vi "Create From VI Reference.vi"(8 "error in (no error)":errorcluster, 10 "VI":refnum<vi>) -> (0 "error out":errorcluster, 3 "CSM-Helper.lvclass":refnum<class "CSM-Helper.lvclass">)   [LabVIEW 2020, in "CSM-Helper.lvclass"]
uses:
  CSM-Helper.lvclass
  CSM-Helper.lvclass/CSM-Helper.ctl
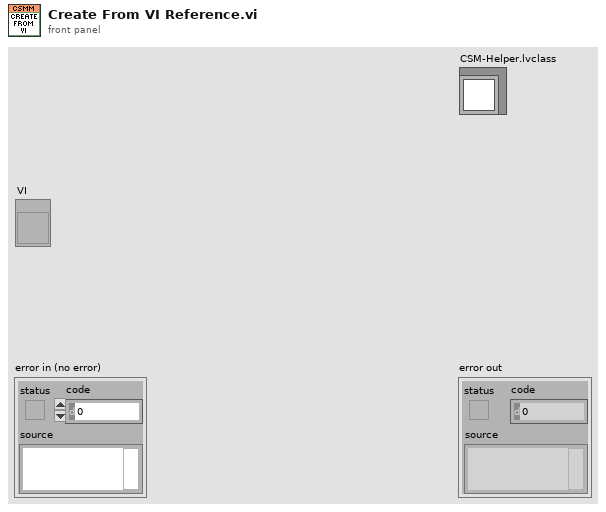
[diagram p1: front panel]
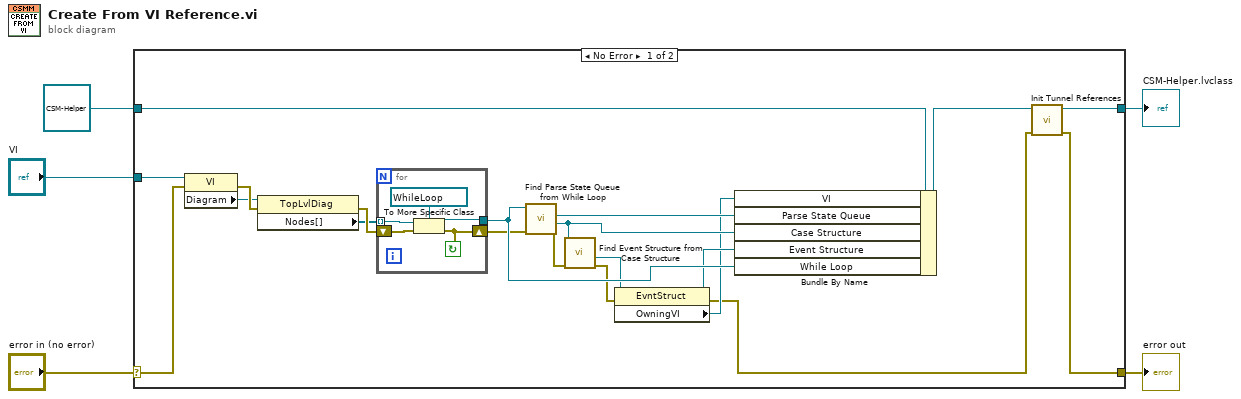
[diagram p0: block diagram]
diagram:
  n1 = case shown="No Error" "error in (no error)" {
    selector: "error in (no error)" -> [w20 w32]
    tunnel: [w6 w32] -> w4
    tunnel: [w8 w31] -> w2
    tunnel: refnum<class "CSM-Helper.lvclass"> refnum ("JKI SM") -> [w19 w31]
    tunnel: "VI" -> [w21 _]
    frame No Error {
      n2 = property class="VI"(reference=w21, error in=w20) -> (error out=w25:errorcluster, "Diagram"=w22:refnum<vi>)  [unwired: 1 out]
      n3 = property class="TopLvlDiag"(reference=w22, error in=w25) -> (error out=w24:errorcluster, "Nodes[]"=w23:refnum<vi>[])  [unwired: 1 out]
      n4 = for {
        tunnel: w23 -> [w29] mode=indexing
        tunnel: [w27] -> w16
        shift-right: [w26] -> w15
        shift-left: w24 -> [w28]
        stop <- w26 continue-if-true
        n5 = To More Specific Class(target class=refnum<vi> refnum ("WLoop Refnum"), reference=w29, error in=w28) -> (specific class reference=w27:refnum<vi>, error out=w26:errorcluster)
      }
      n6 = call "Find Parse State Queue from While Loop.vi"("error in (no error)"=w15, "WhileLoop in"=w16) -> ("error out"=w17:errorcluster, "CaseStructure"=w14:refnum<vi>, "Parse State Queue"=w18:refnum<vi>)  [unwired: 7 in]
      n7 = call "Find Event Structure from Case Structure.vi"("error in (no error)"=w17, "CaseStructure"=w14) -> ("error out"=w10:errorcluster, "EvntStruct Refnum"=w13:refnum<vi>)  [unwired: 8 in]
      n8 = property class="EvntStruct"(reference=w13, error in=w10) -> (reference out=w12:refnum<vi>, error out=w7:errorcluster, "OwningVI"=w11:refnum<vi>)
      n9 = Bundle By Name(cluster=w19, "VI"=w11, "Parse State Queue"=w18, "Case Structure"=w14, "Event Structure"=w12, "While Loop"=w16) -> (w9:refnum<class "CSM-Helper.lvclass">)
      n10 = call "Init Tunnel References.vi"("error in (no error)"=w7, "CSM-Helper in"=w9) -> ("error out"=w6:errorcluster, "CSM-Helper out"=w8:refnum<class "CSM-Helper.lvclass">)  [unwired: 8 in]
    }
    frame Error {
    }
  }
  "error out" <- w4
  "CSM-Helper.lvclass" <- w2
